vi "Init.vi"(8 "error in (no error)":errorcluster, 9 "Constant Action Data":string, 10 "HAL GOOP4.lvlib:Instrument Base":refnum<class "Instrument.lvclass">, 11 "Virt Instrs FGen:Virt Waveform Generator in":refnum<class "Virt Waveform Generator.lvclass">) -> (0 "error out":errorcluster, 3 "Virt Instrs FGen:Virt Waveform Generator out":refnum<class "Virt Waveform Generator.lvclass">)   [LabVIEW 2023, in "Virt Instrs FGen.lvlib" / "Virt Waveform Generator.lvclass"]
uses:
  Virt Waveform Generator.lvclass
  Virt Waveform Generator.lvclass/Virt Waveform Generator.ctl
  Virtual Instrument Base/Virt Instr Base.lvclass
  D:/git/HAL/HAL GOOP4/Virtual Instrument Base/Virt Instr Base.lvclass
  D:/git/HAL/HAL GOOP4/FGen/Virtual FGens/Virt Waveform Generator/Virt Waveform Generator.lvclass
  Instrument/Instrument.lvclass
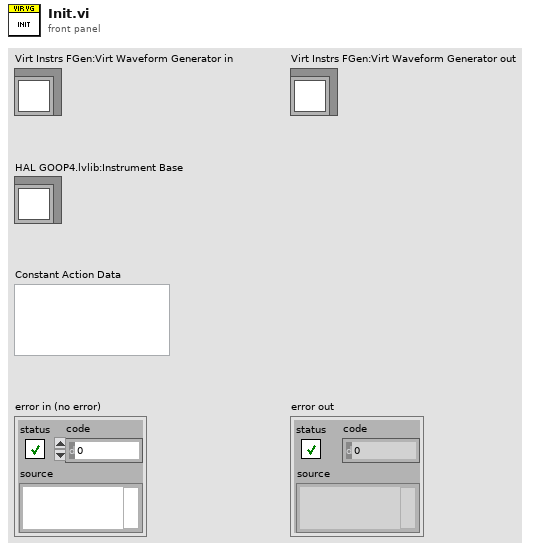
[diagram p1: front panel]
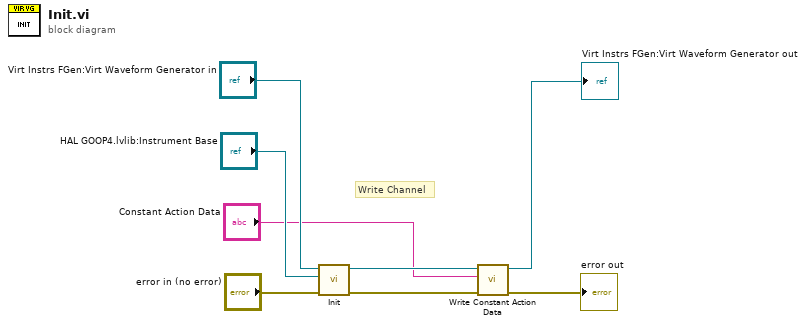
[diagram p0: block diagram]
diagram:
  # "Write Channel"
  n1 = call-parent "Init.vi"("error in (no error)"="error in (no error)", "HAL GOOP4.lvlib:Instrument"="HAL GOOP4.lvlib:Instrument Base", "Virt Instrument Base in"="Virt Instrs FGen:Virt Waveform Generator in") -> ("error out"=w6:errorcluster, "Virt Instrument Base out"=w4:refnum<class "Virt Waveform Generator.lvclass">)  [unwired: 7 in]
  n2 = call "Write Constant Action Data.vi"("error in (no error)"=w6, "Constant Action Data"="Constant Action Data", "Virt Instrument Base in"=w4) -> ("error out"=→"error out":errorcluster, "Virt Instrument Base out"=→"Virt Instrs FGen:Virt Waveform Generator out":refnum<class "Virt Waveform Generator.lvclass">)  [unwired: 7 in]
